vi "Init DAQs (Out).vi"(8 "error in (no error)":errorcluster) -> (0 "error out":errorcluster, 3 "Channel":refnum<k21>)   [LabVIEW 2017]
uses:
  <vilib>/DAQmx/create/channels.llb/DAQmx Create Channel (AO-Voltage-Basic).vi
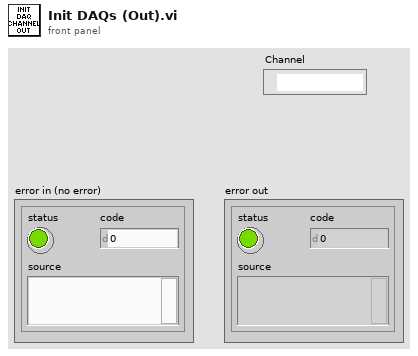
[diagram p1: front panel]
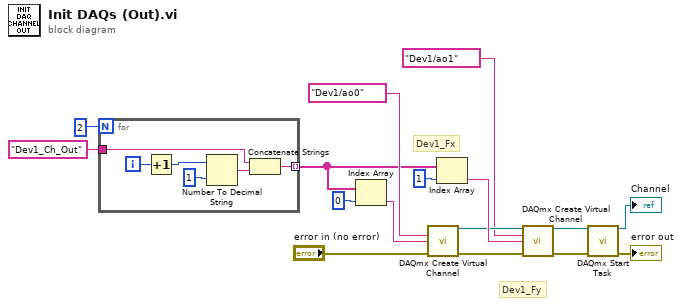
[diagram p0: block diagram]
diagram:
  # "Dev1_Fy"
  # "Dev1_Fx"
  n1 = for {
    N: 2 -> [_]
    tunnel: "Dev1_Ch_Out" ("name to assign") -> [w18]
    tunnel: [w17] -> w3 mode=indexing
    i -> [w22]
    n2 = Increment(x=w22) -> (x+1=w20:i32)
    n3 = Number To Decimal String(number=w20, width (-)=i16 1) -> (decimal integer string=w19:string)
    n4 = Concatenate Strings(w18, w19) -> (w17:string)
  }
  n5 = Index Array(array=w3, index=0) -> (element=w11:string)
  n6 = call-poly <vilib>:"DAQmx Create Virtual Channel.vi"("physical channels"=tag "Dev1/ao0", "name to assign"=w11, "error in"="error in (no error)") -> ("task out"=w7:refnum<k21>, "error out"=w15:errorcluster)  [unwired: 11 in]
  n7 = Index Array(array=w3, index=1) -> (element=w9:string)
  n8 = call-poly <vilib>:"DAQmx Create Virtual Channel.vi"("task in"=w7, "physical channels"=tag "Dev1/ao1", "name to assign"=w9, "error in"=w15) -> ("task out"=w1:refnum<k21>, "error out"=w2:errorcluster)  [unwired: 10 in]
  n9 = call <vilib>:"DAQmx Start Task.vi"("task/channels in"=w1, "error in"=w2) -> ("task out"=→"Channel":refnum<k21>, "error out"=→"error out":errorcluster)  [unwired: 12 in]
